vi "Take_Data_on_the_Move.vi"(3 "Mode":T5, 5 "Traverse line In":T2 {"Carrier_2 Q (l/min)" format="%#.2f"; "Row Duration (mins)" format="%#.1f"; "Row No" min=0; "Trace Gas Concentration (%)" min=0.0 format="%#_4f"; "Carrier_1 Q (l/min)" format="%#.4f"; "Start X" format="%#.2f"; "Start Y" format="%#.2f"; "Start Z" format="%#.2f"; "End X" format="%#.2f"; "End Y" format="%#.2f"; "End Z" format="%#.2f"; "Tunnel Speed" format="%#.2f"; "Averaging time (mins)" min=0.0 format="%#.2f"}) -> (0 "Error Message":string, 1 "Status":T1, 2 "Traverse line Out":T2 {"Carrier_2 Q (l/min)" format="%#.2f"; "Row Duration (mins)" format="%#.1f"; "Row No" min=0; "Trace Gas Concentration (%)" min=0.0 format="%#_4f"; "Carrier_1 Q (l/min)" format="%#.4f"; "Start X" format="%#.2f"; "Start Y" format="%#.2f"; "Start Z" format="%#.2f"; "End X" format="%#.2f"; "End Y" format="%#.2f"; "End Z" format="%#.2f"; "Tunnel Speed" format="%#.2f"; "Averaging time (mins)" min=0.0 format="%#.2f"})   [LabVIEW 2022 SP3]
uses:
  Gen Trav/Traverse_cluster.ctl
  Gen Trav/Spacing.ctl
  Controls/Multi_run_mode.ctl
  Controls/User_Specific_mode.ctl
  Gen Trav/Multi_Run_Status.ctl
  Controls/Save_Data.ctl
  Controls/Setup.ctl
  Globals/Trav_pos_global.vi
  Globals/Preference_global.vi
  Globals/Dynamic_call_global.ph.vi
panel:
  # "X           Y          Z"
  # "Start"
  # "End"
  # "X           Y          Z"
  # "Start"
  # "End"
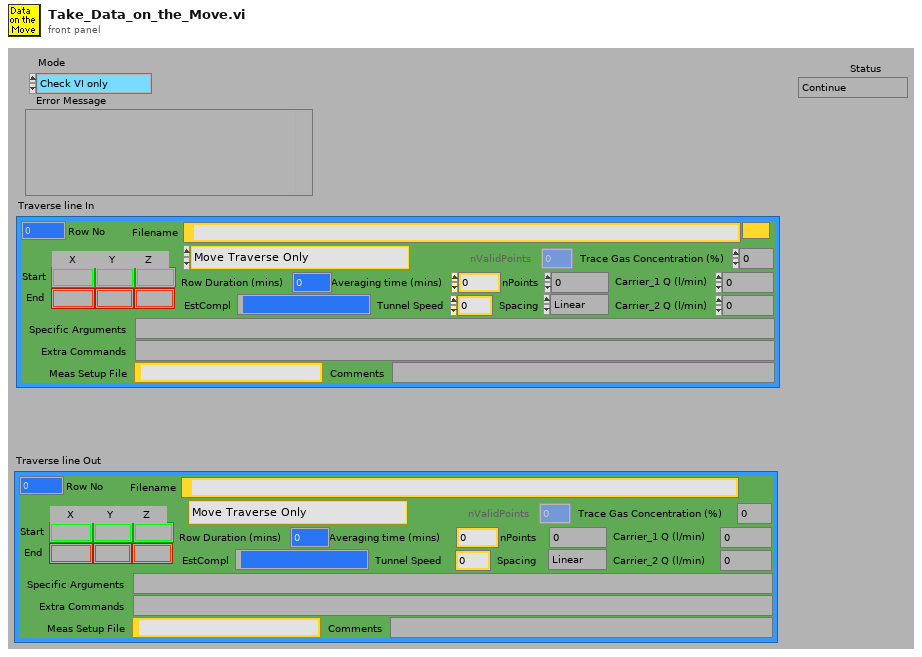
[diagram p1: front panel]
types:
  T1 = typedef "Multi_Run_Status.ctl" = enum16{"Continue", "Continue with Error", "Jump to Next Point", "Jump to Next Row", "Jump To Fall Back", "Terminate Run"}
  T2 = typedef "Traverse_cluster.ctl" = cluster{"Start X":sgl, "Start Y":sgl, "Start Z":sgl, "End X":sgl, "End Y":sgl, "End Z":sgl, "nPoints":i32, "Spacing":T3, "Filename":path, "Tunnel Speed":dbl, "Averaging time (mins)":dbl, "Extra Commands":string, "Carrier_1 Q (l/min)":dbl, "Carrier_2 Q (l/min)":dbl, "Trace Gas Concentration (%)":dbl, "Specific Arguments":string, "Comments":string, "Row No":i32, "Row Type Selector":T4, "EstCompl":string, "Row Duration (mins)":dbl, "nValidPoints":i32, "Meas Setup File":string}
  T3 = typedef "Spacing.ctl" = enum16{"Linear", "Log", "Gauss", "Specified", "N/A"}
  T4 = typedef "Multi_run_mode.ctl" = enum16{"Move Traverse Only", "Set Tunnel Speed Only", "Set Source Only", "Set Measurement Conditions", "Single Measurement", "Vertical Profile", "Lateral Profile", "Longitudinal Profile", "Multi-Axis Profile", "Explore Volume", "Auto Calibrate", "Meas Fast FID Bkgnd", "Check Beam Power", "Scanning Valve Measurement", "Run VI Named:", "Set ADAM Ch", "Wait (minutes)", "Send Message", "Synchronize With:", "Fall Back to this Row", "Turn Off Row Repeating", "Traverse 3D Volume", "Blank Row", "Jump to Fall Back Row"}
  T5 = typedef "User_Specific_mode.ctl" = enum16{"Check VI only", "Run VI"}
  T6 = typedef "Setup.ctl" = enum16{"Run Program", "Show Setup", "Save Current Setup", "Setup Front Panel"}
  T7 = typedef "Save_Data.ctl" = enum16{"Save No Data", "Save Data"}
  T8 = typedef "GMU Gas Line Name.ctl" = enum16{"GMU1 Source", "GMU2 Source", "GMU2 Calib", "CPP GRC-A", "CPP GRC-B"}
  T9 = typedef "Status_Cluster.ctl" = cluster{"Status":T1, "Error Type":string, "Error Description":string}
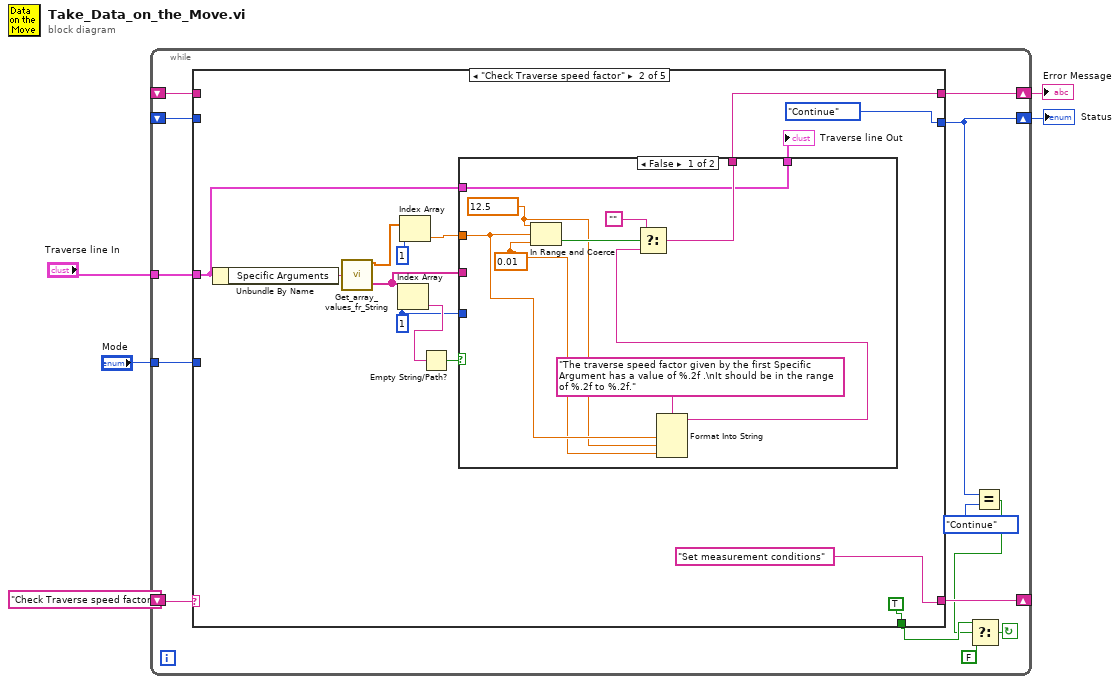
[diagram p0: block diagram]
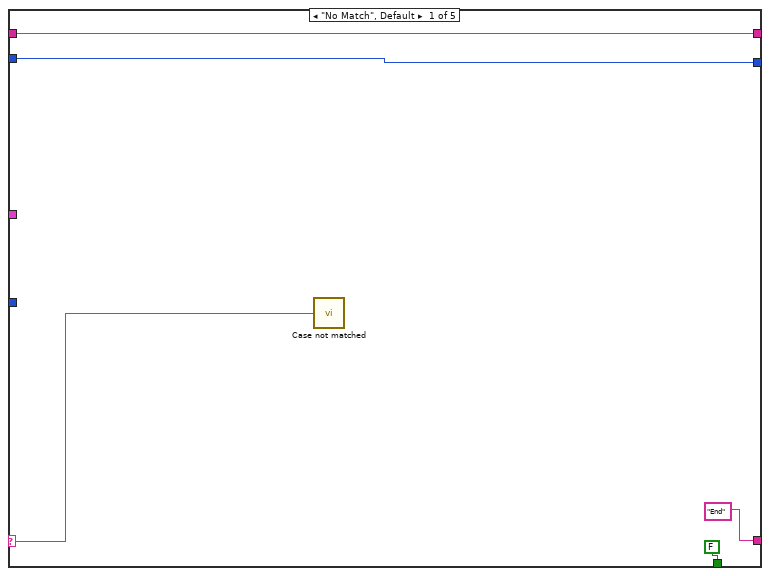
[diagram p2: hidden frame]
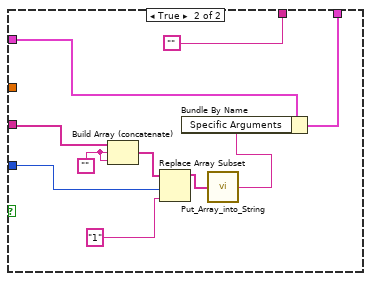
[diagram p3: hidden frame]
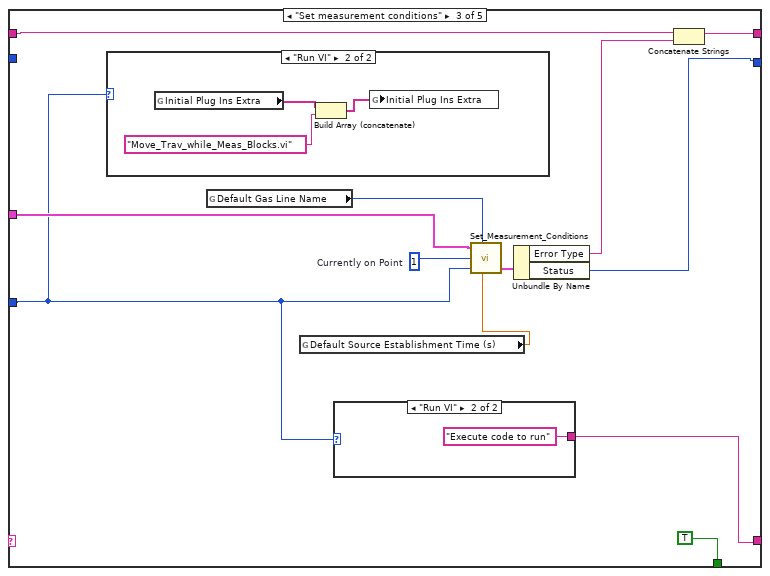
[diagram p4: hidden frame]
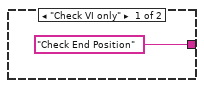
[diagram p6: hidden frame]
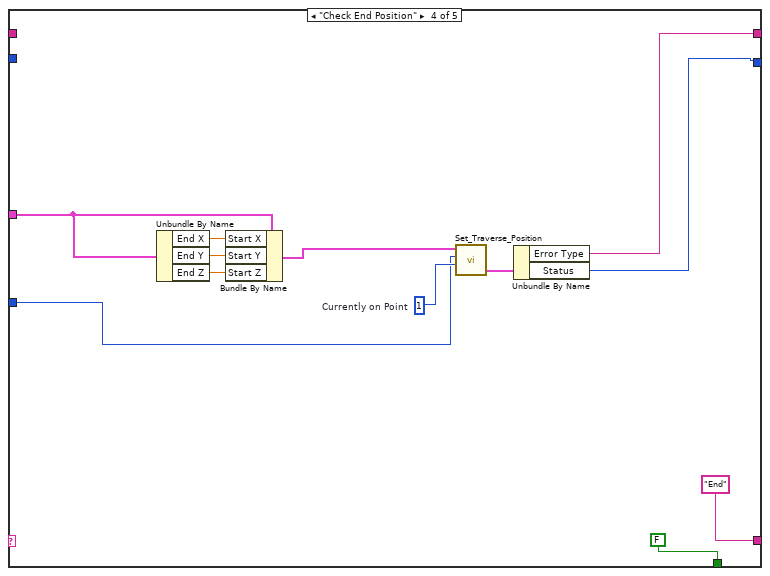
[diagram p7: hidden frame]
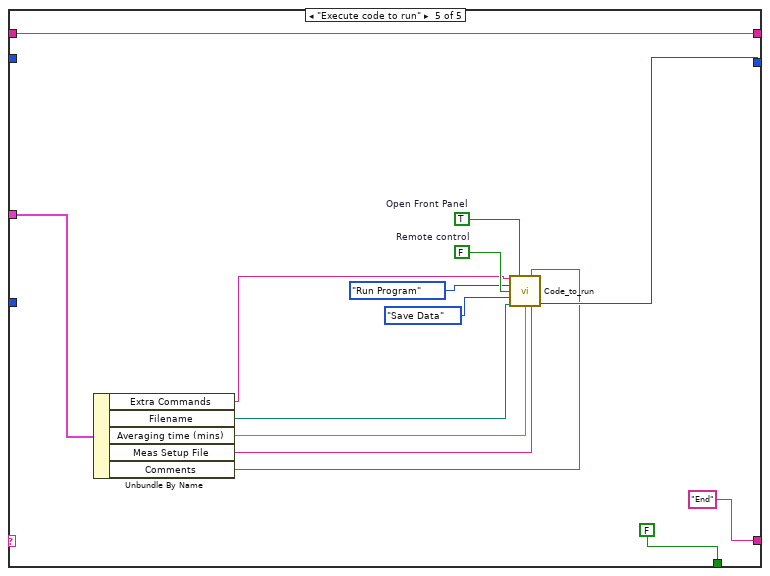
[diagram p8: hidden frame]
diagram:
  n1 = while {
    shift-left: _ -> [w13]
    shift-right: [w8] -> w2
    shift-left: _ -> [w16]
    shift-right: [w14] -> w3
    tunnel: "Traverse line In" -> [w17]
    tunnel: "Mode" -> [w18]
    shift-left: "Check Traverse speed factor" -> [w15]
    shift-right: [w12] -> _
    stop <- w6 continue-if-true
    n2 = case shown="\"Check Traverse speed factor\"" w15 {
      selector: w15 -> [w19 _ _ _ _]
      tunnel: w17 -> [_ w31 w65 w85 w93]
      tunnel: w18 -> [_ _ w57 w77 _]
      tunnel: [FALSE ("Update Datum Powers?") TRUE ("Update Datum Powers?") TRUE ("Update Datum Powers?") FALSE ("Update Datum Powers?") FALSE ("Update Datum Powers?")] -> w11
      tunnel: ["End" "Set measurement conditions" w61 "End" "End"] -> w12
      tunnel: w16 -> [w23 _ w63 _ w92]
      tunnel: [w23 w25 w62 w74 w92] -> w14
      tunnel: w13 -> [w20 _ _ _ _]
      tunnel: [w20 Multi_Run_Status."Continue" ("Status") w66 w83 w96] -> w8
      frame "No Match", Default {
        n3 = call "Case not matched.vi"("Case Name not Matched"=w19) -> ()
      }
      frame "Check Traverse speed factor" {
        w28 = 1 ("index")
        n4 = Unbundle By Name(w31) -> ("Specific Arguments"=w37:string)
        n5 = call "Get_array_values_fr_String.vi"("String Value"=w37) -> ("Numeric Array"=w36:dbl[], "String array"=w27:string[])
        n6 = Index Array(array=w27, index=w28) -> (element=w30:string)
        n7 = Index Array(array=w36, index=1) -> (element=w34:dbl)
        n8 = Empty String/Path?(string/path=w30) -> (empty?=w29:bool)
        n9 = case shown="False" w29 {
          tunnel: w34 -> [w44 _]
          tunnel: [w39 ""] -> w25
          tunnel: [w38 w50] -> w32
          tunnel: w31 -> [w38 w51]
          tunnel: w28 -> [_ w54]
          tunnel: w27 -> [_ w49]
          frame False {
            w42 = 0.01 ("lower limit")
            w43 = 12.5 ("upper limit")
            n10 = In Range and Coerce(upper limit=w43, x=w44, lower limit=w42) -> (In Range?=w46:bool)  [unwired: 1 out]
            n11 = Format Into String(format string="The traverse speed factor given by the first Specific Argument has a value of %.2f .\nIt should be in the range of %.2f to %.2f.", w44, w43, w42) -> (resulting string=w40:string)  [unwired: 2 in, 1 out]
            n12 = Select(t="", s=w46, f=w40) -> (s? t:f=w39:string)
          }
          frame True {
            w48 = ""
            n13 = Build Array (concatenate)(w49, w48, w48) -> (w47:string[])
            n14 = Replace Array Subset(array=w47, new element="1" ("new element/subarray"), index=w54) -> (w55:string[])
            n15 = call "Put_Array_into_String.vi"("String array"=w55) -> ("String Value"=w52:string)
            n16 = Bundle By Name(cluster=w51, "Specific Arguments"=w52) -> (w50:T2)
          }
        }
        "Traverse line Out" <- w32
      }
      frame "Set measurement conditions" {
        w68 = 1  # Currently on Point
        n17 = case shown="\"Run VI\"" w57 {
          frame "Check VI only" {
          }
          frame "Run VI" {
            n18 = global read "Dynamic_call_global.ph.vi" "Initial Plug Ins Extra"() -> (w71:string[])
            n19 = Build Array (concatenate)(w71, "Move_Trav_while_Meas_Blocks.vi") -> (w69:string[])
            n20 = global write "Dynamic_call_global.ph.vi" "Initial Plug Ins Extra"(w69) -> ()
          }
        }
        n21 = global read "Trav_pos_global.vi" "Default Gas Line Name"() -> (w59:T8)
        n22 = global read "Preference_global.vi" "Default Source Establishment Time (s)"() -> (w58:dbl)
        n23 = case shown="\"Run VI\"" w57 {
          tunnel: ["Check End Position" "Execute code to run"] -> w61
          frame "Check VI only" {
          }
          frame "Run VI" {
          }
        }
        n24 = call "Set_Measurement_Conditions.vi"("Traverse line"=w65, "Gas Line Name"=w59, "Currently on Point"=w68, "Simulate/Run"=w57, "Source Establishment Time (s)"=w58) -> ("Status Cluster"=w67:T9)  [unwired: 2 in]
        n25 = Unbundle By Name(w67) -> ("Error Type"=w64:string, "Status"=w66:T1)
        n26 = Concatenate Strings(w63, w64) -> (w62:string)
      }
      frame "Check End Position" {
        w78 = 1  # Currently on Point
        n27 = Unbundle By Name(w85) -> ("End X"=w82:sgl, "End Y"=w81:sgl, "End Z"=w80:sgl)
        n28 = Bundle By Name(cluster=w85, "Start X"=w82, "Start Y"=w81, "Start Z"=w80) -> (w76:T2)
        n29 = call "Set_Traverse_Position.vi"("Currently on Point"=w78, "Simulate/Run"=w77, "Traverse line"=w76) -> ("Status Cluster"=w75:T9)  [unwired: 3 in]
        n30 = Unbundle By Name(w75) -> ("Error Type"=w74:string, "Status"=w83:T1)
      }
      frame "Execute code to run" {
        w97 = TRUE  # Open Front Panel
        w99 = FALSE  # Remote control
        n31 = Unbundle By Name(w93) -> ("Extra Commands"=w88:string, "Filename"=w89:path, "Averaging time (mins)"=w98:dbl, "Meas Setup File"=w87:string, "Comments"=w86:string)
        n32 = call "Code_to_run.vi"("Extra command String"=w88, "Open Front Panel"=w97, "Current Row Comments"=w86, "setup"=Setup."Run Program", "Remote control"=w99, "File"=Save_Data."Save Data", "Results Filename"=w89, "Averaging time (min)"=w98, "Setup filename"=w87) -> ("Status"=w96:T1)  [unwired: 3 in, 3 out]
      }
    }
    n33 = Equal?(x=w8, y=Multi_Run_Status."Continue" ("Status")) -> (x = y?=w10:bool)
    n34 = Select(t=w11, s=w10, f=FALSE) -> (s? t:f=w6:bool)
  }
  "Status" <- w2
  "Error Message" <- w3
